vi "AutoFastPivot.vi"(9 "Heading":dbl, 11 "Pivot Speed":dbl) -> (2 "Finished?":bool)   [LabVIEW 2014]
uses:
  Drivetrain Code/Drivetrain Control.ctl
  Drivetrain Code/Drivetrain Mode.ctl
  Robot Global Data.vi
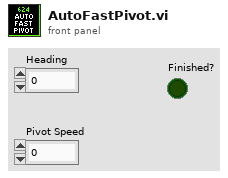
[diagram p1: front panel]
types:
  T1 = typedef "Drivetrain Mode.ctl" = enum16{"Manual", "Gyro Steer", "Vision Steer", "Drive Distance", "Yaw Rate Compensate"}
  T2 = typedef "Drivetrain Control.ctl" = cluster{"Mode":T1, "Steer":dbl, "Y":dbl, "Heading Target":dbl, "Strafe X":dbl, "Y Target":dbl, "Strafe Target":dbl, "X Max Speed":dbl, "X Min Speed":dbl, "Y Max Speed":dbl, "Y Min Speed":dbl, "Force strafe":bool, "Pivot Speed":dbl}
  T3 = typedef "Drivetrain Status.ctl" = cluster{"Y (Throttle)":sgl, "X (Steer)":sgl, "Translation X":sgl, "Center Wheel Down":bool, "Mode":T1, "Distance Drive finished?":bool, "Y Target":sgl, "X Target":sgl, "Heading Target":sgl, "Dist Drive Status":T4, "Step Eject Lockout":bool, "Gyro In Range?":bool, "Yaw Comp Indicators":T5}
  T4 = typedef "Dist Drive Status.ctl" = cluster{"Y In Range":bool, "X In Range":bool, "Gyro In Range":bool, "Y Dist":dbl, "X Dist":dbl, "Gyro":dbl}
  T5 = typedef "Yaw Rate Compensation Indicators.ctl" = cluster{"Rate Command":sgl, "Rate Actual":sgl, "Steer adjustment":sgl}
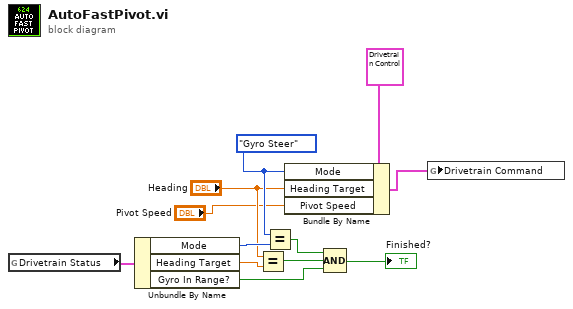
[diagram p0: block diagram]
diagram:
  w9 = Drivetrain_Mode."Gyro Steer" ("Mode")
  n1 = global read "Robot Global Data.vi" "Drivetrain Status"() -> (w10:T3)
  n2 = Unbundle By Name(w10) -> ("Mode"=w8:T1, "Heading Target"=w7:sgl, "Gyro In Range?"=w5:bool)
  n3 = Equal?(x="Heading", y=w7) -> (x = y?=w4:bool)
  n4 = Equal?(x=w9, y=w8) -> (x = y?=w3:bool)
  n5 = Bundle By Name(cluster=T2 {"Mode"=enum."Gyro Steer", "Steer"=0.0, "Y"=0.0, "Heading Target"=0.0, "Strafe X"=0.0, "Y Target"=0.0, "Strafe Target"=0.0, "X Max Speed"=0.0, "X Min Speed"=0.0, "Y Max Speed"=0.0, "Y Min Speed"=0.0, "Force strafe"=FALSE, "Pivot Speed"=0.0} ("Drivetrain Command"), "Mode"=w9, "Heading Target"="Heading", "Pivot Speed"="Pivot Speed") -> (w11:T2)
  n6 = Compound Arithmetic op=AND(w3, w4, w5) -> (→"Finished?":bool)
  n7 = global write "Robot Global Data.vi" "Drivetrain Command"(w11) -> ()
